vi "OpenClose gRPC Connection.vi"(7 "gRPC Connection Action":T2, 8 "error in":errorcluster, 9 "certificatePath":string, 10 "address":string, 11 "gRPC ID In":T1) -> (0 "error out":errorcluster, 3 "gRPC ID Out":T1)   [LabVIEW 2023, in "ThermotronDriverService_Client_Wrapper.lvlib"]
uses:
  ThermotronDriverService_Client_Wrapper.lvlib
  <vilib>/gRPC/LabVIEW gRPC Library/Shared/grpcId.ctl
  <vilib>/ADAS Replay HIL/NodeGrpcService/NodeGrpcService_Client_Wrapper/gRPC Connection Action.ctl
  <vilib>/ADAS Replay HIL/NodeGrpcService/NodeGrpcService_client/NodeGrpcService_client.lvlib
  ThermotronDriverService_client/ThermotronDriverService_client.lvlib
  <vilib>/gRPC/LabVIEW gRPC Library/grpc-lvsupport-release.lvlib
  <vilib>/ADAS Replay HIL/NodeGrpcService/NodeGrpcService_Client_Wrapper/NodeGrpcService_Client_Wrapper.lvlib
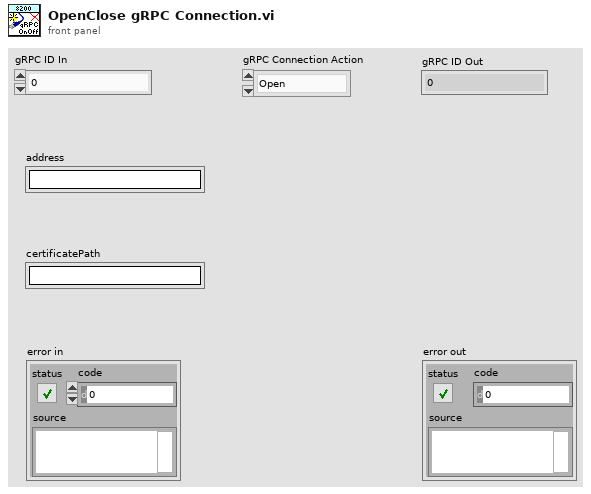
[diagram p1: front panel]
types:
  T1 = typedef "grpc-lvsupport-release.lvlib/grpcId.ctl" = u64
  T2 = typedef "NodeGrpcService_Client_Wrapper.lvlib/gRPC Connection Action.ctl" = enum16{"Open", "Close"}
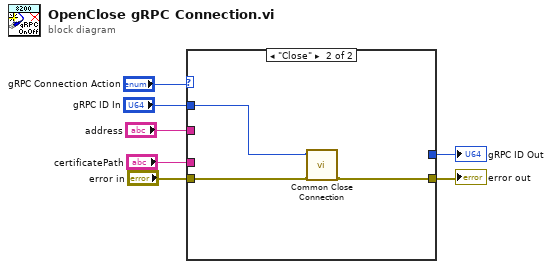
[diagram p0: block diagram]
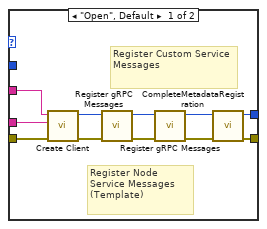
[diagram p2: hidden frame]
diagram:
  n1 = case shown="\"Close\"" "gRPC Connection Action" {
    tunnel: "error in" -> [w18 w20]
    tunnel: "address" -> [w17 _]
    tunnel: "certificatePath" -> [w16 _]
    tunnel: [w15 w19] -> w4
    tunnel: [w14 _] -> w3
    tunnel: "gRPC ID In" -> [_ w21]
    frame "Open", Default {
      # "Register Custom Service Messages"
      # "Register Node Service Messages (Template)"
      n2 = call <vilib>:"Create Client.vi"("error in"=w18, "certificatePath"=w16, "address"=w17) -> ("error out"=w13:errorcluster, "ClientID out"=w12:T1)  [unwired: 7 in]
      n3 = call <vilib>:"Register gRPC Messages.vi"("error in (no error)"=w13, "gRPC ID"=w12) -> ("error out"=w9:errorcluster, "gRPC ID Out"=w10:T1)  [unwired: 8 in]
      n4 = call <vilib>:"Register gRPC Messages.vi"("error in (no error)"=w9, "gRPC ID"=w10) -> ("error out"=w8:errorcluster, "gRPC ID Out"=w11:T1)  [unwired: 8 in]
      n5 = call <vilib>:"CompleteMetadataRegistration.vi"("error in"=w8, "gRPC ID in"=w11) -> ("error out"=w15:errorcluster, "gRPC ID Out"=w14:T1)  [unwired: 8 in]
    }
    frame "Close" {
      n6 = call <vilib>:"Common Close Connection.vi"("error in"=w20, "gRPC ID"=w21) -> ("error out"=w19:errorcluster)  [unwired: 9 in]
    }
  }
  "error out" <- w4
  "gRPC ID Out" <- w3
